vi "Pre Launch Init.vi"(11 "SinglePhotonInterferenceUI in":refnum<class "SinglePhotonInterferenceUI.lvclass">) -> (0 "error out":errorcluster, 3 "SinglePhotonInterferenceUI out":refnum<class "SinglePhotonInterferenceUI.lvclass">)   [LabVIEW 2023, in "SinglePhotonInterferenceUI.lvlib" / "SinglePhotonInterferenceUI.lvclass"]
doc: "(<B>Filename</B>: Actor Framework.lvlib:Actor.lvclass:Pre Launch Init.vi)\n\nDefines behavior that occurs after the Launch Nested Actor method is invoked but before the actor's Actor Core method begins running.\n\nBy default, this method does nothing. A descendant class may override it to define behavior."
uses:
  SinglePhotonInterferenceUI.lvclass
  <vilib>/ActorFramework/Actor/Actor.lvclass
  CountsHistos.ctl
  typedefs/typedefs.lvlib
  ConcreteClasses/ConcreteInstrumentClasses/Multiharp/Multiharp/_lib/PQ/MultiHarp/MH_InitInfo.ctl
panel:
  in  "MH Init Done":cluster{"DevIdx":i32, "Init Info":T1}
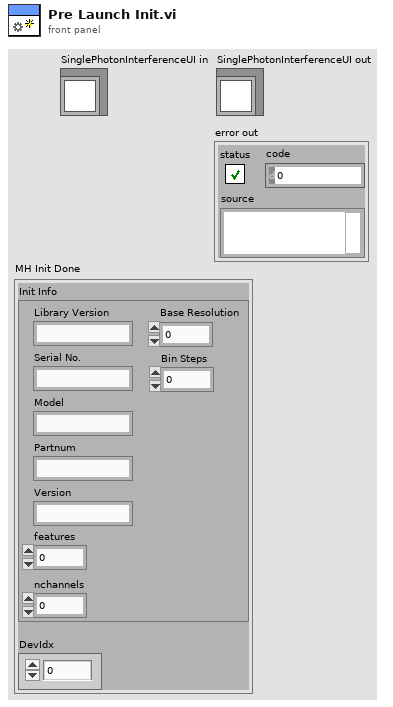
[diagram p1: front panel]
types:
  T1 = typedef "typedefs.lvlib/MH_InitInfo.ctl" = cluster{"Library Version":string, "Serial No.":string, "Model":string, "Partnum":string, "Version":string, "features":i32, "nchannels":i32, "Base Resolution":dbl, "Bin Steps":i32}
  T2 = cluster{"MH_Meas_Error":errorcluster, "Coincidences":i32[]}
  T3 = typedef "typedefs.lvlib/CountsHistos.ctl" = cluster{"cntrates":i32[], "syncrate":i32, "Histograms":u32[], "ActualHistoLe":i32}
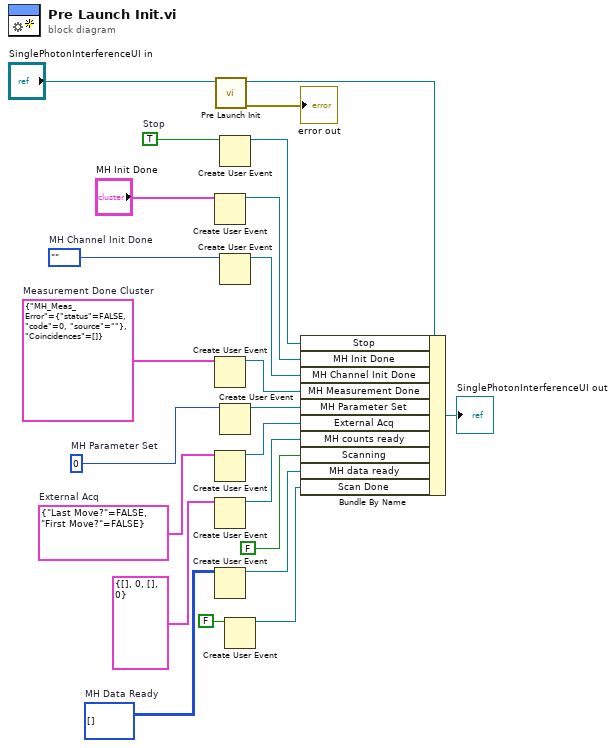
[diagram p0: block diagram]
diagram:
  w3 = T2 {"MH_Meas_Error"={"status"=FALSE, "code"=0, "source"=""}, "Coincidences"=[]}  # Measurement Done Cluster
  w5 = cluster{"Last Move?":bool, "First Move?":bool} {"Last Move?"=FALSE, "First Move?"=FALSE}  # External Acq
  w11 = i32[][] []  # MH Data Ready
  w13 = enum16{""}.""  # MH Channel Init Done
  w19 = 0  # MH Parameter Set
  w20 = TRUE  # Stop
  n1 = Create User Event(user event datatype="MH Init Done") -> (user event=w18:refnum<user-event>)  [unwired: 1 in, 1 out]
  n2 = Create User Event(user event datatype=w3) -> (user event=w16:refnum<user-event>)  [unwired: 1 in, 1 out]
  n3 = Create User Event(user event datatype=w5) -> (user event=w4:refnum<user-event>)  [unwired: 1 in, 1 out]
  n4 = Create User Event(user event datatype=T3 {"cntrates"=[], "syncrate"=0, "Histograms"=[], "ActualHistoLe"=0} ("Counts")) -> (user event=w7:refnum<user-event>)  [unwired: 1 in, 1 out]
  n5 = Create User Event(user event datatype=w11) -> (user event=w9:refnum<user-event>)  [unwired: 1 in, 1 out]
  n6 = call-parent "Pre Launch Init.vi"("Actor in"="SinglePhotonInterferenceUI in") -> ("error out"=→"error out":errorcluster, "Actor out"=w12:refnum<class "SinglePhotonInterferenceUI.lvclass">)  [unwired: 9 in]
  n7 = Create User Event(user event datatype=w20) -> (user event=w21:refnum<user-event>)  [unwired: 1 in, 1 out]
  n8 = Create User Event(user event datatype=w13) -> (user event=w15:refnum<user-event>)  [unwired: 1 in, 1 out]
  n9 = Create User Event(user event datatype=w19) -> (user event=w17:refnum<user-event>)  [unwired: 1 in, 1 out]
  n10 = Create User Event(user event datatype=FALSE ("Scanning")) -> (user event=w2:refnum<user-event>)  [unwired: 1 in, 1 out]
  n11 = Bundle By Name(cluster=w12, "Stop"=w21, "MH Init Done"=w18, "MH Channel Init Done"=w15, "MH Measurement Done"=w16, "MH Parameter Set"=w17, "External Acq"=w4, "MH counts ready"=w7, "Scanning"=FALSE, "MH data ready"=w9, "Scan Done"=w2) -> (→"SinglePhotonInterferenceUI out":refnum<class "SinglePhotonInterferenceUI.lvclass">)
